vi "Parse Average IG Pressure.vi"(11 "Buffer in":string) -> (2 "mean":dbl, 3 "Buffer out":string)   [LabVIEW 2019, in "PGC2D.lvlib"]
uses:
  PGC2D.lvlib
  <vilib>/Analysis/baseanly.llb/Mean (DBL).vi
  <vilib>/Analysis/NI_AALBase.lvlib
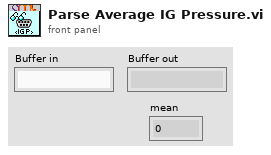
[diagram p1: front panel]
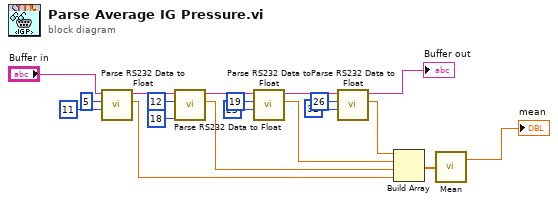
[diagram p0: block diagram]
diagram:
  n1 = call "Parse RS232 Data to Float.vi"("AML end byte"=11, "AML start byte"=5, "bytes in"="Buffer in") -> ("DBL data"=w15:dbl, "bytes out"=w12:string)  [unwired: 7 in]
  n2 = call "Parse RS232 Data to Float.vi"("AML end byte"=18, "AML start byte"=12, "bytes in"=w12) -> ("DBL data"=w17:dbl, "bytes out"=w13:string)  [unwired: 7 in]
  n3 = call "Parse RS232 Data to Float.vi"("AML end byte"=25, "AML start byte"=19, "bytes in"=w13) -> ("DBL data"=w16:dbl, "bytes out"=w14:string)  [unwired: 7 in]
  n4 = call "Parse RS232 Data to Float.vi"("AML end byte"=32, "AML start byte"=26, "bytes in"=w14) -> ("DBL data"=w18:dbl, "bytes out"=→"Buffer out":string)  [unwired: 7 in]
  n5 = Build Array(w18, w16, w17, w15) -> (w3:dbl[])
  n6 = call-poly <vilib>:"Mean.vi"("X"=w3) -> ("mean"=→"mean":dbl)  [unwired: 1 out]
